vi "CLD 16 state machine solution.vi"() -> ()   [LabVIEW 2009]
doc: "CLD-Übung 16\n\nDieses VI enthält hauptsächlich die Fälle der Ereignisstruktur. Die Verwendung von Eigenschaftsknoten zum Aktivieren und Deaktivieren von Eigenschaften ist eine gängige Praxis."
uses:
  CLD 16 Control Panel.ctl
  CLD 16 Status Panel.ctl
  CLD 16 Data Cluster.ctl
  CLD 16 state enum.ctl
panel:
  out "Produktionsstrecke 2 aktiv":bool
  out "Produktionsstrecke 1 aktiv":bool
  out "Fehler (Ausgang)":T1
  in  "Fehler (Eingang)":T1
  in  "Stopp-Schaltfläche":bool
  in  "Systemsteuerung - Produktionsstrecke 2":T2
  out "Prozesssteuerung":T3 {"Prozesswert" format="%#.3g"}
  in  "Systemsteuerung - Produktionsstrecke 1":T2
  # "Anzeigepanel"
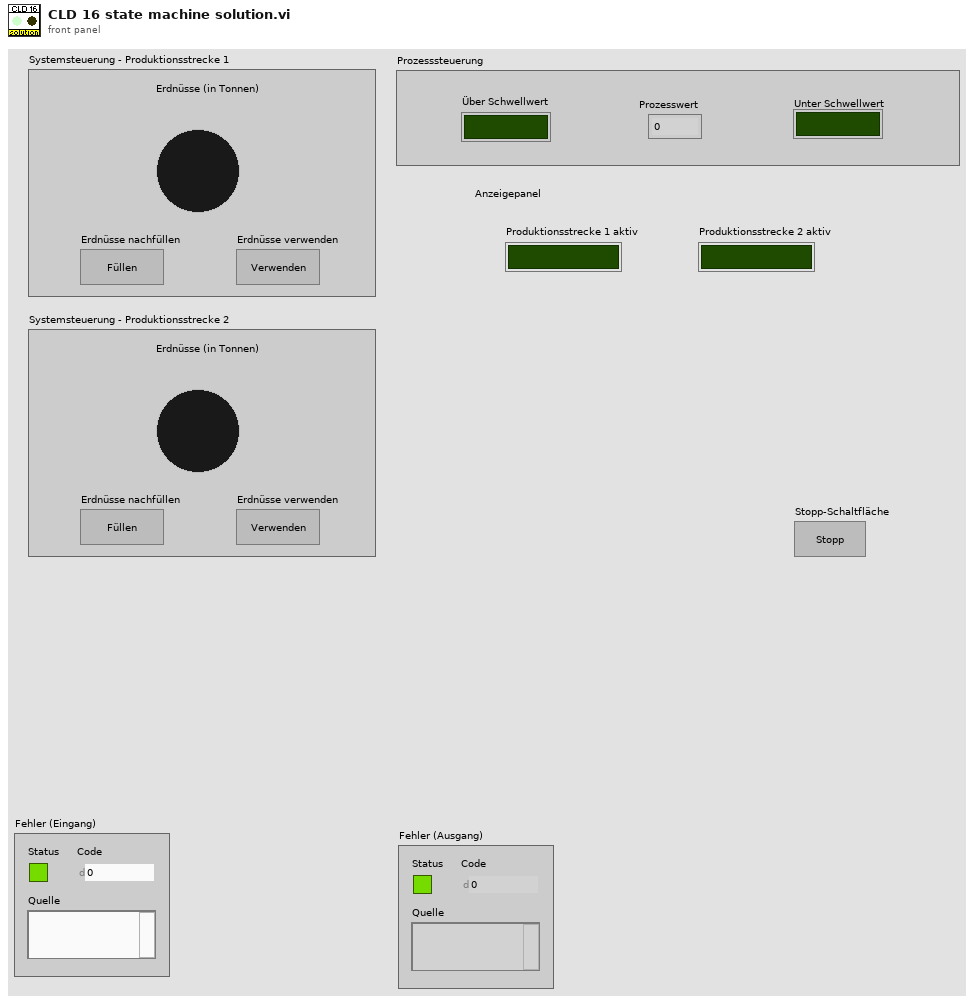
[diagram p1: front panel]
types:
  T1 = cluster{"Status":bool, "Code":i32, "Quelle":string}
  T2 = typedef "CLD 16 Control Panel.ctl" = cluster{"Erdnüsse (in Tonnen)":i8, "Erdnüsse nachfüllen":bool, "Erdnüsse verwenden":bool}
  T3 = typedef "CLD 16 Status Panel.ctl" = cluster{"Über Schwellwert":bool, "Unter Schwellwert":bool, "Prozesswert":dbl}
  T4 = typedef "CLD 16 Data Cluster.ctl" = cluster{"Systemsteuerungs-Array":T2[], "Statusanzeige":T3, "Produktionsstrecke 1":bool, "Produktionsstrecke 2":bool, "Stopp-Schaltfläche":bool}
  T5 = typedef "CLD 16 state enum.ctl" = enum16{"Initialisieren", "Verwenden", "Ruhezustand"}
  T6 = enum8{"Enabled", "Disabled", "Disabled and Grayed Out"}
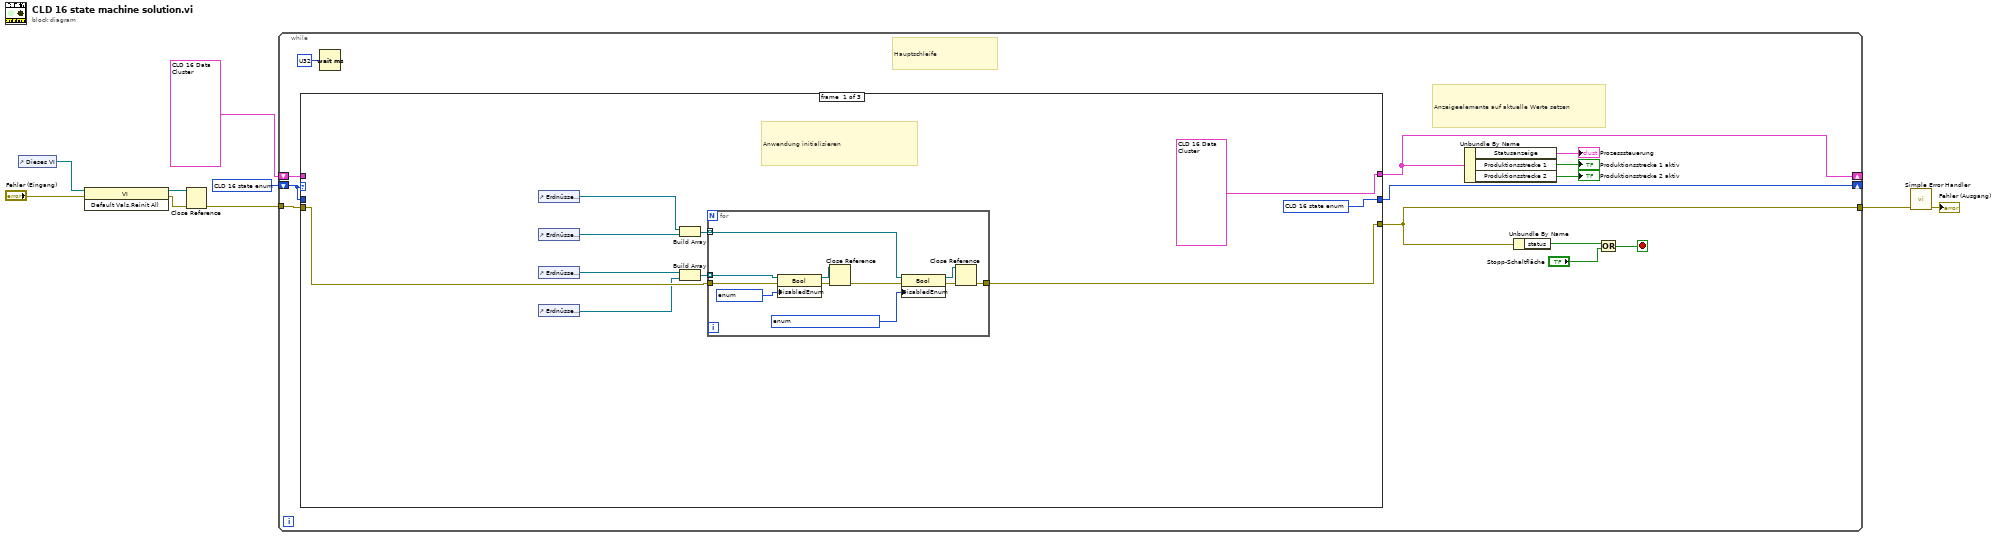
[diagram p0: block diagram]
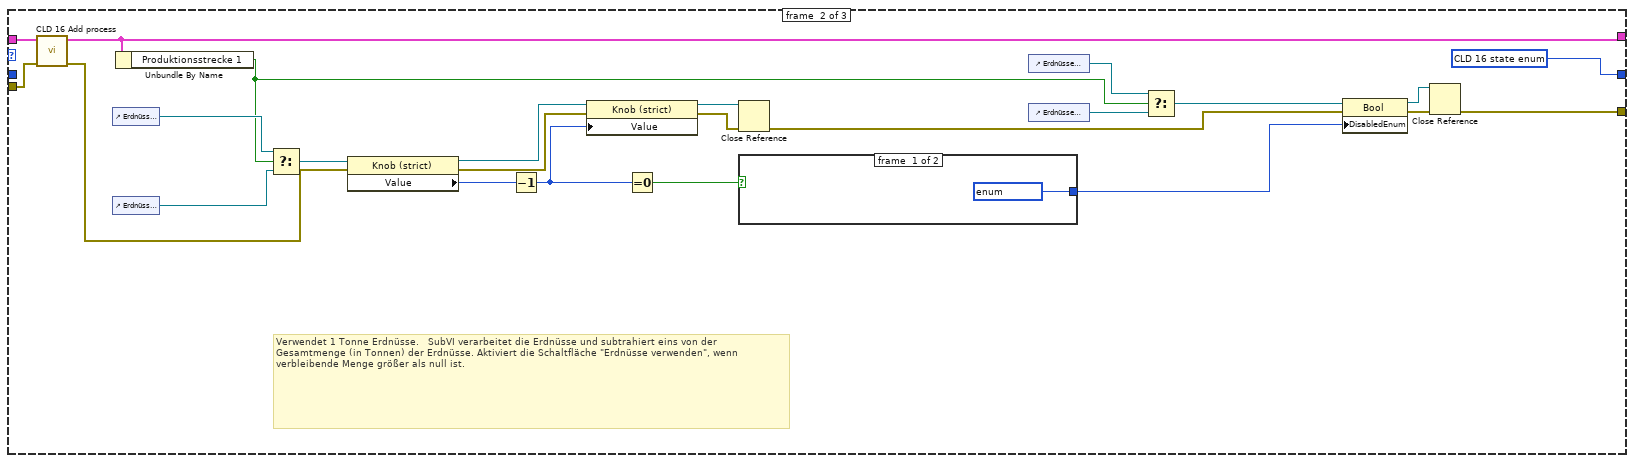
[diagram p2: hidden frame]
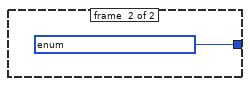
[diagram p3: hidden frame]
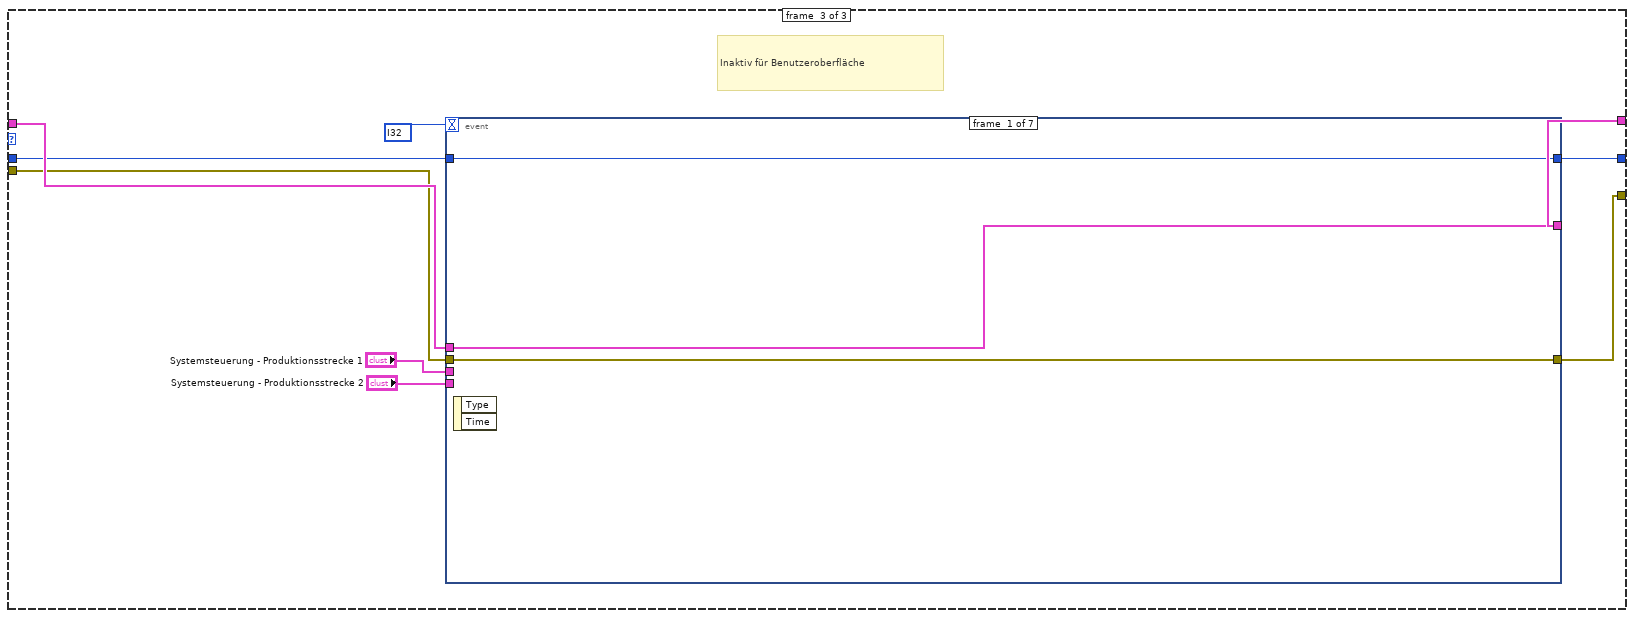
[diagram p4: hidden frame]
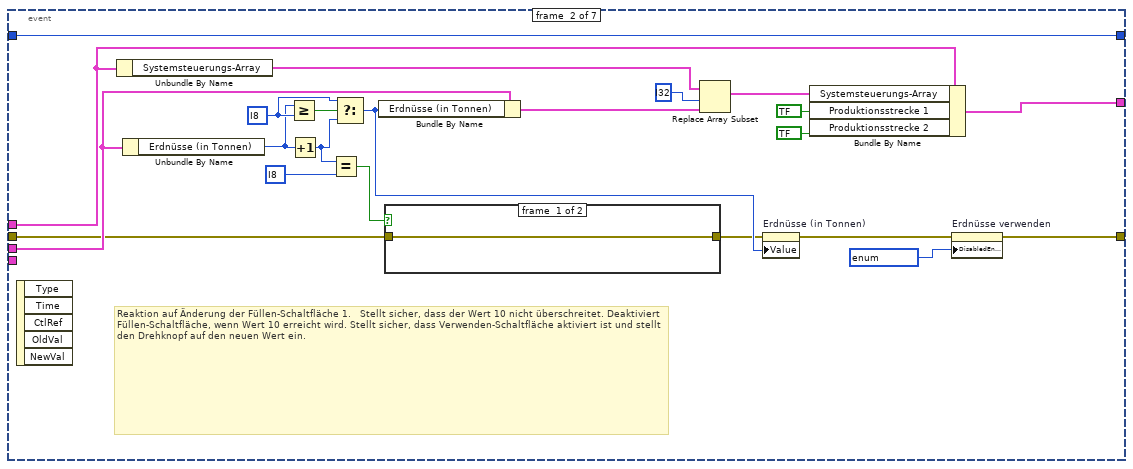
[diagram p5: hidden frame]
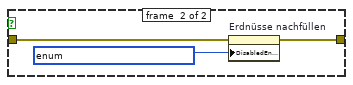
[diagram p6: hidden frame]
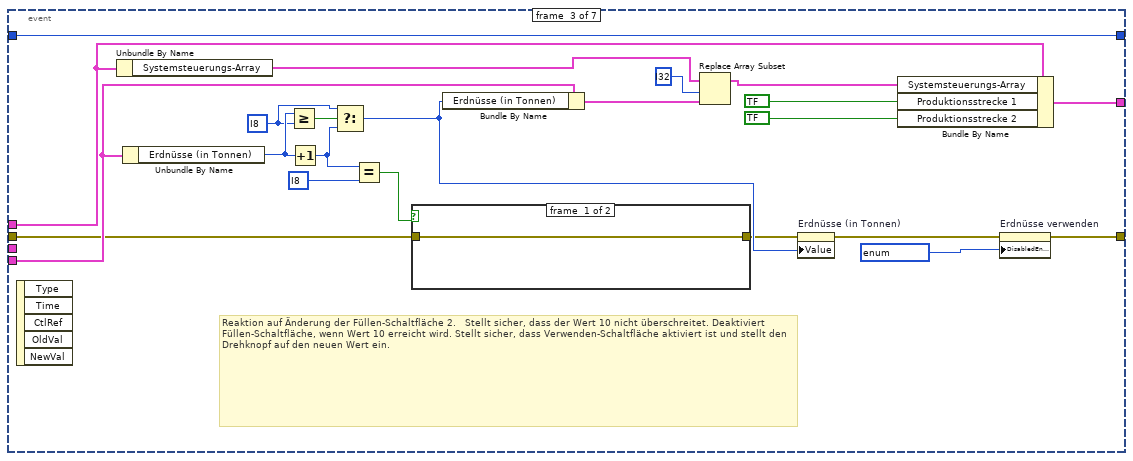
[diagram p7: hidden frame]
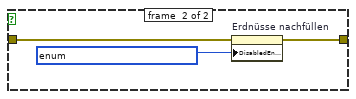
[diagram p8: hidden frame]
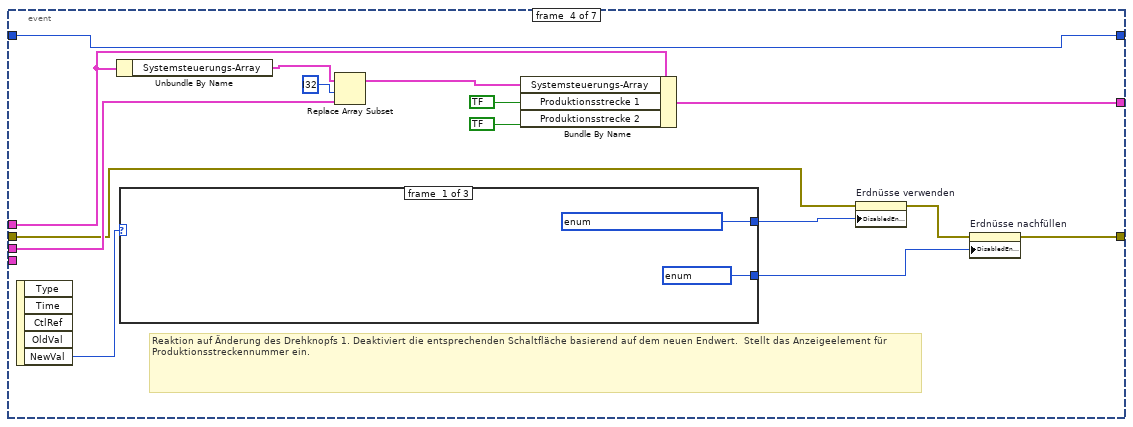
[diagram p9: hidden frame]
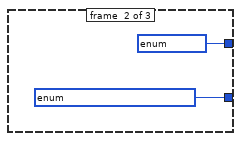
[diagram p10: hidden frame]
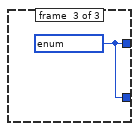
[diagram p11: hidden frame]
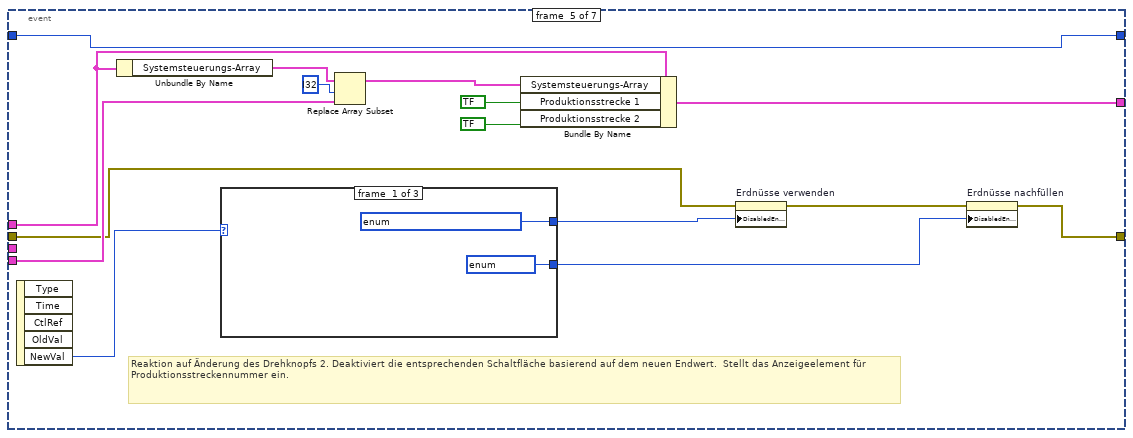
[diagram p12: hidden frame]
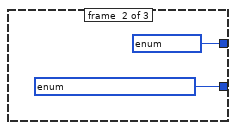
[diagram p13: hidden frame]
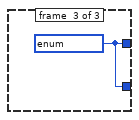
[diagram p14: hidden frame]
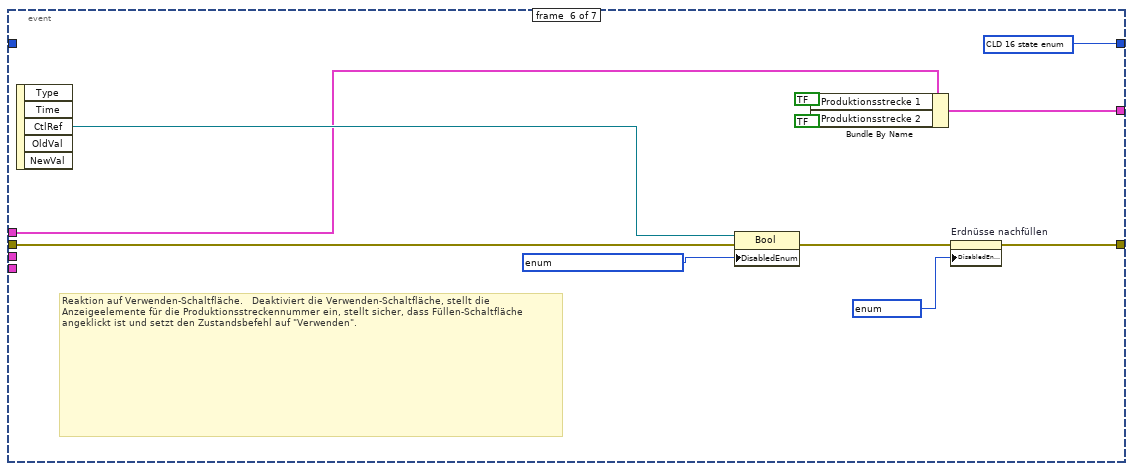
[diagram p15: hidden frame]
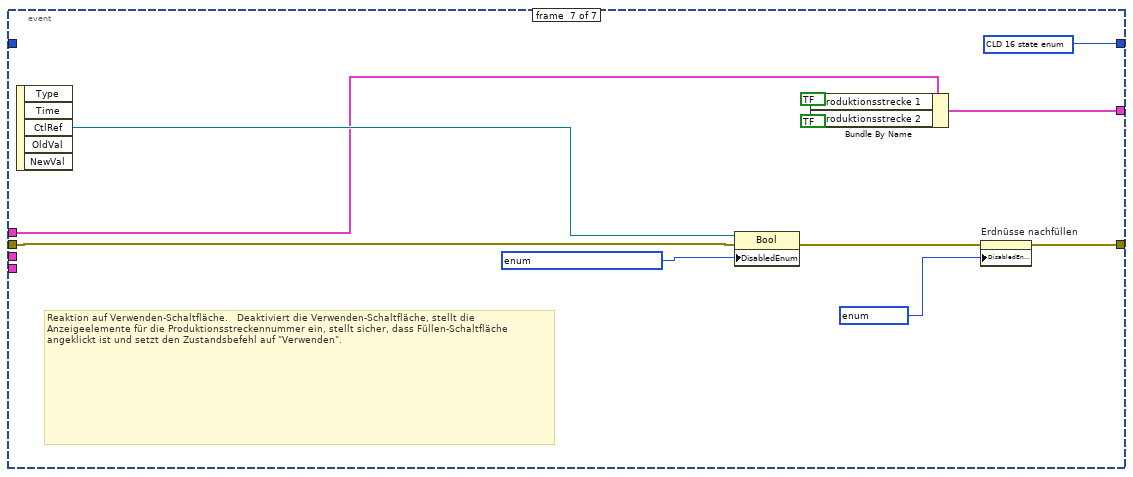
[diagram p16: hidden frame]
diagram:
  n1 = control-ref of="Dieses VI"() -> (w4:refnum<vi>)
  n2 = invoke on="Invoke Node" class="VI" method="Default Vals.Reinit All"(reference=w4, error in="Fehler (Eingang)") -> (reference out=w2:refnum<vi>, error out=w5:errorcluster)  [unwired: 1 in, 1 out]
  n3 = Close Reference(reference=w2, error in (no error)=w5) -> (error out=w3:errorcluster)
  n4 = while {
    shift-right: [w21] -> _
    shift-left: T5 ? ("CLD 16 - Zustände") -> [w22]
    shift-right: [w14] -> _
    shift-left: T4 ? ("Cluster") -> [w20]
    tunnel: [w18] -> w8
    tunnel: w3 -> [w19]
    stop <- w17 stop-if-true
    # "Hauptschleife"
    # "Anzeigeelemente auf aktuelle Werte setzen"
    n5 = case shown="\"Ruhezustand\", Default" w22 {
      tunnel: [T5 ? ("CLD 16 - Zustände") T5 ? ("CLD 16 - Zustände") w73] -> w21
      tunnel: w22 -> [_ _ w74]
      tunnel: w20 -> [_ w67 w78]
      tunnel: [T4 ? ("Cluster") w65 w77] -> w14
      tunnel: [w27 w46 w70] -> w18
      tunnel: w19 -> [w28 w45 w71]
      frame #0 {
        # "Anwendung initialisieren"
        n6 = control-ref of="Erdnüsse verwenden"() -> (w30:refnum<vi>)
        n7 = control-ref of="Erdnüsse verwenden"() -> (w29:refnum<vi>)
        n8 = control-ref of="Erdnüsse nachfüllen"() -> (w25:refnum<vi>)
        n9 = control-ref of="Erdnüsse nachfüllen"() -> (w24:refnum<vi>)
        n10 = Build Array(w30, w29) -> (w31:refnum<vi>[])
        n11 = Build Array(w25, w24) -> (w23:refnum<vi>[])
        n12 = for {
          tunnel: w31 -> [w40] mode=indexing
          tunnel: w28 -> [w37]
          tunnel: [w39] -> w27
          tunnel: w23 -> [w38] mode=indexing
          n13 = property on="Property Node" class="Bool"(reference=w38, error in=w37, "DisabledEnum"=T6 ? ("Deaktiviert")) -> (reference out=w33:refnum<vi>, error out=w36:errorcluster)
          n14 = Close Reference(reference=w33, error in (no error)=w36) -> (error out=w34:errorcluster)
          n15 = property on="Property Node" class="Bool"(reference=w40, error in=w34, "DisabledEnum"=T6 ? ("Deaktiviert")) -> (reference out=w42:refnum<vi>, error out=w43:errorcluster)
          n16 = Close Reference(reference=w42, error in (no error)=w43) -> (error out=w39:errorcluster)
        }
      }
      frame #1 {
        # "Verwendet 1 Tonne Erdnüsse.   SubVI verarbeitet die Erdnüsse und subtrahiert eins von der Gesamtmenge (in Tonnen) der Erdnüsse. Aktiviert die Schaltfläche \"Erdnüsse verwenden\", wenn verbleibende Menge größer als null ist."
        n17 = call "CLD 16 Add process.vi"("Fehler (Eingang, kein Fehler)"=w45, "Cluster (Eingang)"=w67) -> ("Fehler (Ausgang)"=w44:errorcluster, "Cluster (Ausgang)"=w65:T4)  [unwired: 8 in]
        n18 = control-ref of="Erdnüsse (in Tonnen)"() -> (w57:refnum<vi>)
        n19 = control-ref of="Erdnüsse (in Tonnen)"() -> (w58:refnum<vi>)
        n20 = Unbundle By Name(w65) -> ("Produktionsstrecke 1"=w56:bool)
        n21 = Select(t=w57, s=w56, f=w58) -> (s? t:f=w54:refnum<vi>)
        n22 = property on="Property Node" class="Knob (strict)"(reference=w54, error in=w44) -> (reference out=w53:refnum<vi>, error out=w48:errorcluster, "Value"=w55:i8)
        n23 = Decrement(x=w55) -> (x-1=w50:i8)
        n24 = property on="Property Node" class="Knob (strict)"(reference=w53, error in=w48, "Value"=w50) -> (reference out=w51:refnum<vi>, error out=w52:errorcluster)
        n25 = Equal To 0?(x=w50) -> (x = 0?=w49:bool)
        n26 = Close Reference(reference=w51, error in (no error)=w52) -> (error out=w47:errorcluster)
        n27 = case shown="True" w49 {
          tunnel: [T6 ? ("Deaktiviert") T6 ? ("Deaktiviert")] -> w62
          frame #0 {
          }
          frame #1 {
          }
        }
        n28 = control-ref of="Erdnüsse verwenden"() -> (w64:refnum<vi>)
        n29 = control-ref of="Erdnüsse verwenden"() -> (w61:refnum<vi>)
        n30 = Select(t=w64, s=w56, f=w61) -> (s? t:f=w63:refnum<vi>)
        n31 = property on="Property Node" class="Bool"(reference=w63, error in=w47, "DisabledEnum"=w62) -> (reference out=w59:refnum<vi>, error out=w60:errorcluster)
        n32 = Close Reference(reference=w59, error in (no error)=w60) -> (error out=w46:errorcluster)
      }
      frame #2 {
        # "Inaktiv für Benutzeroberfläche"
        n33 = event shown="[5] \"Systemsteuerung - Produktionsstrecke 1.Erdnüsse verwenden\": Value Change" {
          selector: _ -> [_ _ _ _ _ _ _]
          dyn-events: _ -> [_ _ _ _ _ _ _]
          timeout: i32 ? -> [_ _ _ _ _ _ _]
          tunnel: w78 -> [w80 w102 w128 w147 w167 w179 w190]
          tunnel: [w80 w103 w129 w148 w168 w178 w189] -> w77
          tunnel: "Systemsteuerung - Produktionsstrecke 1" -> [_ w95 _ w140 _ _ _]
          tunnel: [w81 w98 w124 w143 w163 T5 ? ("CLD 16 - Zustände") T5 ? ("CLD 16 - Zustände")] -> w73
          tunnel: w74 -> [w81 w98 w124 w143 w163 _ _]
          tunnel: "Systemsteuerung - Produktionsstrecke 2" -> [_ _ w115 _ w158 _ _]
          tunnel: w71 -> [w79 w90 w114 w137 w157 w177 w188]
          tunnel: [w79 w88 w112 w135 w155 w175 w186] -> w70
          event #0 {
            n34 = event-data() -> ()  [unwired: 1 in, 2 out]
          }
          event #1 {
            w91 = i8 ? ("x")
            # "Reaktion auf Änderung der Füllen-Schaltfläche 1.   Stellt sicher, dass der Wert 10 nicht überschreitet. Deaktiviert Füllen-Schaltfläche, wenn Wert 10 erreicht wird. Stellt sicher, dass Verwenden-Schaltfläche aktiviert ist und stellt den Drehknopf auf den neuen Wert ein."
            n35 = event-data() -> ()  [unwired: 1 in, 5 out]
            n36 = Unbundle By Name(w102) -> ("Systemsteuerungs-Array"=w101:T2[])
            n37 = Unbundle By Name(w95) -> ("Erdnüsse (in Tonnen)"=w83:i8)
            n38 = Greater Or Equal?(x=w83, y=w91) -> (x >= y?=w86:bool)
            n39 = Increment(x=w83) -> (x+1=w82:i8)
            n40 = Equal?(x=w82, y=i8 ? ("x")) -> (x = y?=w84:bool)
            n41 = Select(t=w91, s=w86, f=w82) -> (s? t:f=w92:i8)
            n42 = Bundle By Name(cluster=w95, "Erdnüsse (in Tonnen)"=w92) -> (w94:T2)
            n43 = case shown="True" w84 {
              tunnel: w90 -> [w104 w107]
              tunnel: [w104 w106] -> w87
              frame #0 {
              }
              frame #1 {
                n44 = property on="Erdnüsse nachfüllen" class="Bool"(error in=w107, "DisabledEnum"=T6 ? ("Deaktiviert")) -> (error out=w106:errorcluster)  [unwired: 1 in, 1 out]
              }
            }
            n45 = Replace Array Subset(array=w101, new element=w94, index=i32 ? ("Index")) -> (w99:T2[])
            n46 = property on="Erdnüsse (in Tonnen)" class="Knob (strict)"(error in=w87, "Value"=w92) -> (error out=w89:errorcluster)  [unwired: 1 in, 1 out]
            n47 = Bundle By Name(cluster=w102, "Systemsteuerungs-Array"=w99, "Produktionsstrecke 1"=bool ?, "Produktionsstrecke 2"=bool ? ("Produktionsstrecke 1")) -> (w103:T4)
            n48 = property on="Erdnüsse verwenden" class="Bool"(error in=w89, "DisabledEnum"=T6 ? ("Deaktiviert")) -> (error out=w88:errorcluster)  [unwired: 1 in, 1 out]
          }
          event #2 {
            w116 = i8 ? ("x")
            # "Reaktion auf Änderung der Füllen-Schaltfläche 2.   Stellt sicher, dass der Wert 10 nicht überschreitet. Deaktiviert Füllen-Schaltfläche, wenn Wert 10 erreicht wird. Stellt sicher, dass Verwenden-Schaltfläche aktiviert ist und stellt den Drehknopf auf den neuen Wert ein."
            n49 = event-data() -> ()  [unwired: 1 in, 5 out]
            n50 = Unbundle By Name(w128) -> ("Systemsteuerungs-Array"=w127:T2[])
            n51 = Unbundle By Name(w115) -> ("Erdnüsse (in Tonnen)"=w117:i8)
            n52 = Greater Or Equal?(x=w117, y=w116) -> (x >= y?=w119:bool)
            n53 = Increment(x=w117) -> (x+1=w110:i8)
            n54 = Select(t=w116, s=w119, f=w110) -> (s? t:f=w118:i8)
            n55 = Equal?(x=w110, y=i8 ? ("x")) -> (x = y?=w108:bool)
            n56 = case shown="True" w108 {
              tunnel: w114 -> [w130 w133]
              tunnel: [w130 w132] -> w109
              frame #0 {
              }
              frame #1 {
                n57 = property on="Erdnüsse nachfüllen" class="Bool"(error in=w133, "DisabledEnum"=T6 ? ("Deaktiviert")) -> (error out=w132:errorcluster)  [unwired: 1 in, 1 out]
              }
            }
            n58 = Bundle By Name(cluster=w115, "Erdnüsse (in Tonnen)"=w118) -> (w121:T2)
            n59 = Replace Array Subset(array=w127, new element=w121, index=i32 ? ("Index")) -> (w125:T2[])
            n60 = property on="Erdnüsse (in Tonnen)" class="Knob (strict)"(error in=w109, "Value"=w118) -> (error out=w113:errorcluster)  [unwired: 1 in, 1 out]
            n61 = Bundle By Name(cluster=w128, "Systemsteuerungs-Array"=w125, "Produktionsstrecke 1"=bool ?, "Produktionsstrecke 2"=bool ? ("Produktionsstrecke 1")) -> (w129:T4)
            n62 = property on="Erdnüsse verwenden" class="Bool"(error in=w113, "DisabledEnum"=T6 ? ("Deaktiviert")) -> (error out=w112:errorcluster)  [unwired: 1 in, 1 out]
          }
          event #3 {
            # "Reaktion auf Änderung des Drehknopfs 1. Deaktiviert die entsprechenden Schaltfläche basierend auf dem neuen Endwert.  Stellt das Anzeigeelement für Produktionsstreckennummer ein."
            n63 = event-data() -> ("NewVal"=w138:i8)  [unwired: 1 in, 4 out]
            n64 = Unbundle By Name(w147) -> ("Systemsteuerungs-Array"=w146:T2[])
            n65 = case shown="10" w138 {
              tunnel: [T6 ? ("Deaktiviert") T6 ? ("Deaktiviert") w153] -> w139
              tunnel: [T6 ? ("Deaktiviert") T6 ? ("Deaktiviert") w153] -> w134
              frame #0 {
              }
              frame #1 {
              }
              frame #2 {
                w153 = T6 ? ("Deaktiviert")
              }
            }
            n66 = Replace Array Subset(array=w146, new element=w140, index=i32 ? ("Index")) -> (w144:T2[])
            n67 = Bundle By Name(cluster=w147, "Systemsteuerungs-Array"=w144, "Produktionsstrecke 1"=bool ?, "Produktionsstrecke 2"=bool ? ("Produktionsstrecke 1")) -> (w148:T4)
            n68 = property on="Erdnüsse verwenden" class="Bool"(error in=w137, "DisabledEnum"=w139) -> (error out=w136:errorcluster)  [unwired: 1 in, 1 out]
            n69 = property on="Erdnüsse nachfüllen" class="Bool"(error in=w136, "DisabledEnum"=w134) -> (error out=w135:errorcluster)  [unwired: 1 in, 1 out]
          }
          event #4 {
            # "Reaktion auf Änderung des Drehknopfs 2. Deaktiviert die entsprechenden Schaltfläche basierend auf dem neuen Endwert.  Stellt das Anzeigeelement für Produktionsstreckennummer ein."
            n70 = event-data() -> ("NewVal"=w159:i8)  [unwired: 1 in, 4 out]
            n71 = Unbundle By Name(w167) -> ("Systemsteuerungs-Array"=w166:T2[])
            n72 = case shown="1..9, Default" w159 {
              tunnel: [T6 ? ("Deaktiviert") T6 ? ("Deaktiviert") w173] -> w160
              tunnel: [T6 ? ("Deaktiviert") T6 ? ("Deaktiviert") w173] -> w154
              frame #0 {
              }
              frame #1 {
              }
              frame #2 {
                w173 = T6 ? ("Deaktiviert")
              }
            }
            n73 = Replace Array Subset(array=w166, new element=w158, index=i32 ? ("Index")) -> (w164:T2[])
            n74 = Bundle By Name(cluster=w167, "Systemsteuerungs-Array"=w164, "Produktionsstrecke 1"=bool ?, "Produktionsstrecke 2"=bool ? ("Produktionsstrecke 1")) -> (w168:T4)
            n75 = property on="Erdnüsse verwenden" class="Bool"(error in=w157, "DisabledEnum"=w160) -> (error out=w156:errorcluster)  [unwired: 1 in, 1 out]
            n76 = property on="Erdnüsse nachfüllen" class="Bool"(error in=w156, "DisabledEnum"=w154) -> (error out=w155:errorcluster)  [unwired: 1 in, 1 out]
          }
          event #5 {
            # "Reaktion auf Verwenden-Schaltfläche.   Deaktiviert die Verwenden-Schaltfläche, stellt die Anzeigeelemente für die Produktionsstreckennummer ein, stellt sicher, dass Füllen-Schaltfläche angeklickt ist und setzt den Zustandsbefehl auf \"Verwenden\"."
            n77 = event-data() -> ("CtlRef"=w183:refnum<vi>)  [unwired: 1 in, 4 out]
            n78 = property on="Property Node" class="Bool"(reference=w183, error in=w177, "DisabledEnum"=T6 ? ("Deaktiviert")) -> (error out=w176:errorcluster)  [unwired: 1 out]
            n79 = Bundle By Name(cluster=w179, "Produktionsstrecke 1"=bool ?, "Produktionsstrecke 2"=bool ? ("Produktionsstrecke 1")) -> (w178:T4)
            n80 = property on="Erdnüsse nachfüllen" class="Bool"(error in=w176, "DisabledEnum"=T6 ? ("Deaktiviert")) -> (error out=w175:errorcluster)  [unwired: 1 in, 1 out]
          }
          event #6 {
            # "Reaktion auf Verwenden-Schaltfläche.   Deaktiviert die Verwenden-Schaltfläche, stellt die Anzeigeelemente für die Produktionsstreckennummer ein, stellt sicher, dass Füllen-Schaltfläche angeklickt ist und setzt den Zustandsbefehl auf \"Verwenden\"."
            n81 = event-data() -> ("CtlRef"=w194:refnum<vi>)  [unwired: 1 in, 4 out]
            n82 = property on="Property Node" class="Bool"(reference=w194, error in=w188, "DisabledEnum"=T6 ? ("Deaktiviert")) -> (error out=w187:errorcluster)  [unwired: 1 out]
            n83 = Bundle By Name(cluster=w190, "Produktionsstrecke 1"=bool ?, "Produktionsstrecke 2"=bool ? ("Produktionsstrecke 1")) -> (w189:T4)
            n84 = property on="Erdnüsse nachfüllen" class="Bool"(error in=w187, "DisabledEnum"=T6 ? ("Deaktiviert")) -> (error out=w186:errorcluster)  [unwired: 1 in, 1 out]
          }
        }
      }
    }
    n85 = Wait (ms)(milliseconds to wait=u32 ? ("Zu wartende ms")) -> ()  [unwired: 1 out]
    n86 = Unbundle By Name(w14) -> ("Statusanzeige"=→"Prozesssteuerung":T3, "Produktionsstrecke 1"=→"Produktionsstrecke 1 aktiv":bool, "Produktionsstrecke 2"=→"Produktionsstrecke 2 aktiv":bool)
    n87 = Unbundle By Name(w18) -> ("status"=w15:bool)
    n88 = Or(x=w15, y="Stopp-Schaltfläche") -> (x .or. y?=w17:bool)
  }
  n89 = call <vilib>:"Simple Error Handler.vi"("error in (no error)"=w8) -> ("error out"=→"Fehler (Ausgang)":errorcluster)  [unwired: 4 in, 4 out]
